vi "LEDS Controller.vi"(8 "error in":errorcluster) -> ()   [LabVIEW 2019]
doc: "This VI executes continuously carrying out the current operation and responding to updates or new operations. It will often contain the timing or control code that is difficult to place directly in TeleOp. This VI generally opens all sensors and motors and isolates the rest of the robot code from knowing how the operations are carried out."
uses:
  <vilib>/Rock Robotics/WPI/Framework/Completion Status.ctl
  LEDS Setpoints.ctl
  LEDS Operations.ctl
  <vilib>/Rock Robotics/SystemInterfaces/DIO/FPGA_DIOPWMChannel.ctl
  <vilib>/Rock Robotics/WPI/MotorControl/WPI_MotorControlOpen SPARK.vi
  <vilib>/Rock Robotics/Network Tables/NT Write Boolean.vi
panel:
  in  "Numeric":dbl=50.0
  in  "Interactive Values":T1={"Operation"=enum."Seizure-inducing", "Setpoint"=0.0, "Duration"=0.0, "seizure active"=FALSE, "pwmOutput"=0.0}
  out "Current\nCmd":string="Started at  17:26:23.947\n: Seizure-inducing,  S 0.0, D 0.000000"
  in  "Buttons":cluster{"Execute Cmd":bool, "Abort Cmd":bool}
  out "Command Timing":cluster{"Start Time (ms)":u32, "Iterations":i32}={"Start Time (ms)"=5015241, "Iterations"=0}
  out "Status":T3
  # "Tip: It may be helpful to observe inputs and sensor values.\nYou may also want to display tuning or debugging controls."
  # "Interactive Command: You may fill in the settings for a command\nand schedule it with the Execute button. You can observe and abort\nany command while fine tuning the code for the controller."
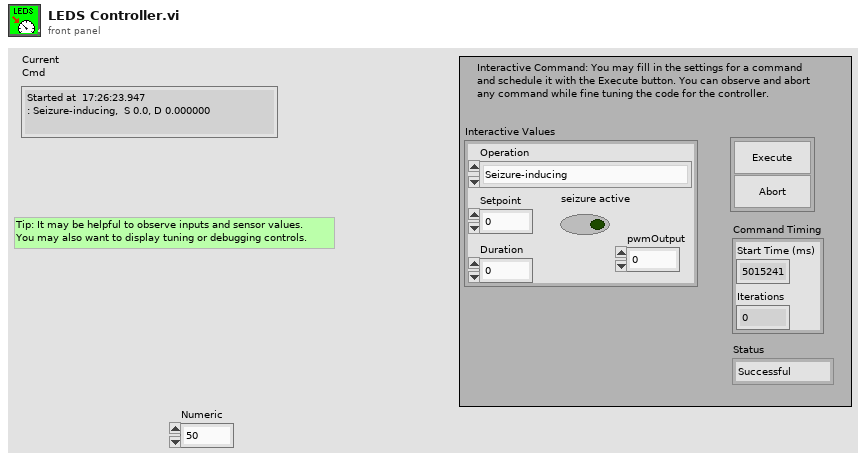
[diagram p1: front panel]
types:
  T1 = typedef "LEDS Setpoints.ctl" = cluster{"Operation":T2, "Setpoint":dbl, "Duration":dbl, "seizure active":bool, "pwmOutput":dbl}
  T2 = typedef "LEDS Operations.ctl" = enum16{"Reserve", "Read Current", "Immediate", "Seizure-inducing"}
  T3 = typedef "Completion Status.ctl" = enum16{"Successful", "Aborted", "Incomplete"}
  T4 = typedef "FPGA_DIOPWMChannel.ctl" = enum8{"PWM 0", "PWM 1", "PWM 2", "PWM 3", "PWM 4", "PWM 5", "PWM 6", "PWM 7", "PWM 8", "PWM 9", "PWM MXP 0", "PWM MXP 1", "PWM MXP 2", "PWM MXP 3", "PWM MXP 4", "PWM MXP 5", "PWM MXP 6", "PWM MXP 7", "PWM MXP 8", "PWM MXP 9", "Invalid"}
  T5 = typedef "WPI_MotorControlDeviceRef.ctl" = cluster{"DeviceStatus":errorcluster, "Type":T6, "PWM":cluster{"PWM Channel":T4, "DeadBand":T7}, "CAN":cluster{"Device Number":u8, "SetOutput VI Ref":variant, "GetOutput VI Ref":variant, "Enable VI Ref":variant, "Disable VI Ref":variant, "Data":variant}, "Invert":bool, "DIO PWM":cluster{"PWM \"Enable\" Channel":T4, "DIOChannel":T8, "PWM Rate":dbl}}
  T6 = typedef "WPI_MotorControlType.ctl" = enum16{"PWM", "CAN", "DIO PWM"}
  T7 = typedef "WPI_PWMDeadband.ctl" = cluster{"Name":string, "maxPositivePwm":i32, "minPositivePwm":i32, "centerPwm":i32, "maxNegativePwm":i32, "minNegativePwm":i32, "angularRange":u16}
  T8 = typedef "FPGA_DIOChannel.ctl" = enum8{"DIO 0", "DIO 1", "DIO 2", "DIO 3", "DIO 4", "DIO 5", "DIO 6", "DIO 7", "DIO 8", "DIO 9", "DIO MXP 0", "DIO MXP 1", "DIO MXP 2", "DIO MXP 3", "DIO MXP 4", "DIO MXP 5", "DIO MXP 6", "DIO MXP 7", "DIO MXP 8", "DIO MXP 9", "DIO MXP 10", "DIO MXP 11", "DIO MXP 12", "DIO MXP 13", "DIO MXP 14", "DIO MXP 15", "SPI Port CS1", "SPI Port CS2", "SPI Port CS3", "SPI Port MISO", "SPI Port MOSI", "Invalid"}
  T9 = typedef "Command Status Info.ctl" = cluster{"Name":string, "Status":T3, "notifier out":T10}
  T10 = typedef "Completion Notifier.ctl" = refnum<notifier>
  T11 = cluster{"Current Command":T1, "Command Timing":cluster{"Start Time (ms)":u32, "Iterations":i32}, "Command Arguments":cluster{"Command Info":T9, "Description":string, "Default Command":T1, "queue out":refnum<queue>, "Subsystem Name":string}}
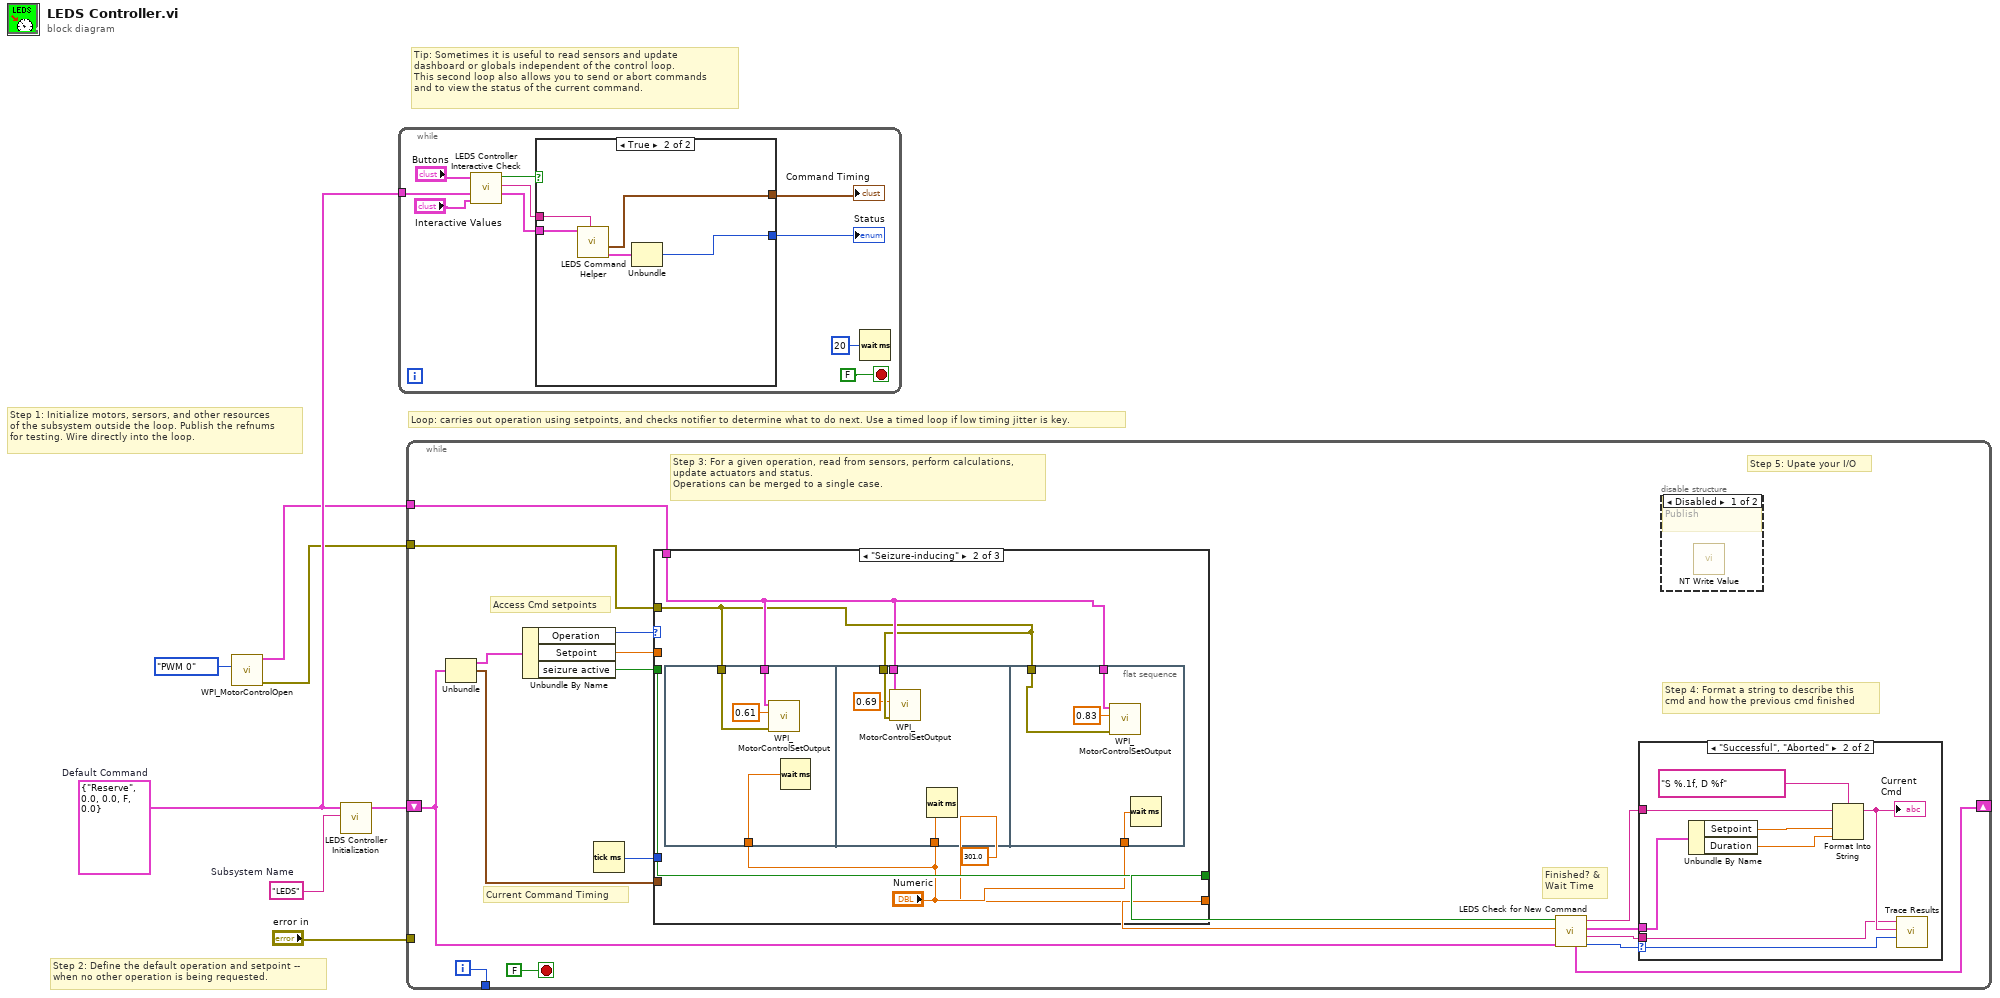
[diagram p0: block diagram]
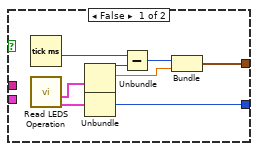
[diagram p2: hidden frame]
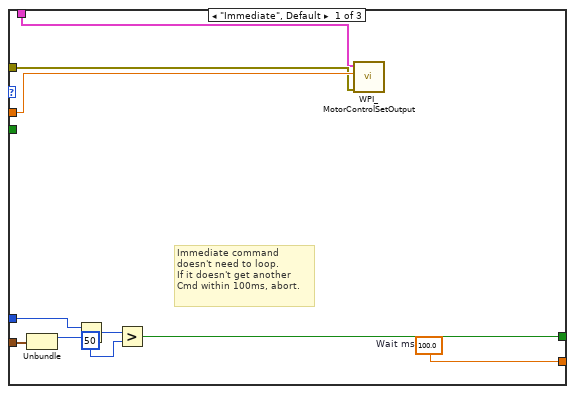
[diagram p5: hidden frame]
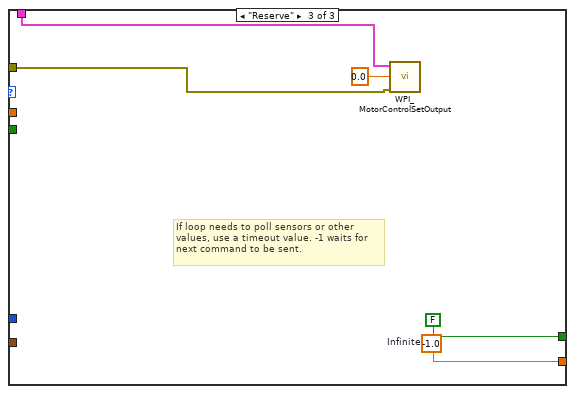
[diagram p6: hidden frame]
diagram:
  w4 = T1 {"Operation"=enum."Reserve", "Setpoint"=0.0, "Duration"=0.0, "seizure active"=FALSE, "pwmOutput"=0.0}  # Default Command
  w5 = "LEDS"  # Subsystem Name
  # "Tip: Sometimes it is useful to read sensors and update\ndashboard or globals independent of the control loop.\nThis second loop also allows you to send or abort commands\nand to view the status of the current command."
  # "Step 2: Define the default operation and setpoint --\nwhen no other operation is being requested."
  # "Step 1: Initialize motors, sersors, and other resources\nof the subsystem outside the loop. Publish the refnums\nfor testing. Wire directly into the loop."
  # "Loop: carries out operation using setpoints, and checks notifier to determine what to do next. Use a timed loop if low timing jitter is key."
  n1 = call-poly <vilib>:"WPI_MotorControlOpen.vi"("PWM Channel"=FPGA_DIOPWMChannel."PWM 0") -> ("error out"=w1:errorcluster, "MotorControlDeviceRef"=w2:T5)  [unwired: 9 in]
  n2 = call "LEDS Controller Initialization.vi"("Subsystem Name"=w5, "Default Command"=w4) -> ("Current Command"=w6:T11)  [unwired: 9 in]
  n3 = while {
    tunnel: w4 -> [w14]
    stop <- FALSE stop-if-true
    n4 = call "LEDS Controller Interactive Check.vi"("Interactive Command in"="Interactive Values", "Default Command"=w14, "Buttons"="Buttons") -> ("Interactive Command out"=w11:T1, "Trace String"=w12:string, "Schedule"=w13:bool)  [unwired: 6 in]
    n5 = case shown="True" w13 {
      tunnel: [w25 w30] -> w10
      tunnel: w11 -> [_ w28]
      tunnel: [w21 w26] -> w9
      tunnel: w12 -> [_ w29]
      frame False {
        n6 = Tick Count (ms)() -> (millisecond timer value=w20:u32)
        n7 = call "Read LEDS Operation.vi"() -> ("Command Info"=w18:T9, "SubSystem Data"=w19:T1)  [unwired: 9 in, 1 out]
        n8 = Unbundle(w19) -> ("Operation"=w24:T2, "Setpoint"=w22:dbl)  [unwired: 3 out]
        n9 = Unbundle(w18) -> ("Status"=w25:T3)  [unwired: 2 out]
        n10 = Subtract(x=w20, y=w24) -> (x-y=w23:u32)
        n11 = Bundle(w23, "Setpoint"=w22) -> (w21:cluster{u32, "Setpoint":dbl})  [unwired: 1 in]
      }
      frame True {
        n12 = call "LEDS Command Helper.vi"("Description"=w29, "SubSystem Data"=w28) -> ("Command Info Out"=w27:T9, "Command Timing"=w26:cluster{"Start Time (ms)":u32, "Iterations":i32})  [unwired: 7 in, 1 out]
        n13 = Unbundle(w27) -> ("Status"=w30:T3)  [unwired: 2 out]
      }
    }
    "Status" <- w10
    "Command Timing" <- w9
    n14 = Wait (ms)(milliseconds to wait=u32 20) -> ()  [unwired: 1 out]
  }
  n15 = while {
    shift-right: [w41] -> _
    shift-left: w6 -> [w34]
    tunnel: [w47] -> _
    tunnel: "error in" -> [_]
    tunnel: w2 -> [w31]
    tunnel: w1 -> [w32]
    i -> [w47]
    stop <- FALSE stop-if-true
    # "Step 5: Upate your I/O"
    # "Step 4: Format a string to describe this\ncmd and how the previous cmd finished"
    # "Current Command Timing"
    # "Access Cmd setpoints"
    # "Finished? &\nWait Time"
    # "Step 3: For a given operation, read from sensors, perform calculations,\nupdate actuators and status.\nOperations can be merged to a single case."
    n16 = Unbundle(w34) -> ("Current Command"=w46:T1, "Command Timing"=w42:cluster{"Start Time (ms)":u32, "Iterations":i32})  [unwired: 1 out]
    n17 = Unbundle By Name(w46) -> ("Operation"=w45:T2, "Setpoint"=w44:dbl, "seizure active"=w33:bool)
    n18 = Tick Count (ms)() -> (millisecond timer value=w43:u32)
    n19 = case shown="\"Seizure-inducing\"" w45 {
      tunnel: [w66 301.0 ("Infinite") w88] -> w39
      tunnel: [w60 w71 FALSE ("ignore previous (F)")] -> w40
      tunnel: w42 -> [w62 _ _]
      tunnel: w44 -> [w59 _ _]
      tunnel: w43 -> [w61 _ _]
      tunnel: w33 -> [_ w71 _]
      tunnel: w32 -> [w58 w67 w84]
      tunnel: w31 -> [w57 w68 w85]
      frame "Immediate", Default {
        w66 = 100.0  # Wait ms
        # "Immediate command\ndoesn't need to loop.\nIf it doesn't get another\nCmd within 100ms, abort."
        n20 = Unbundle(w62) -> ("Start Time (ms)"=w65:u32)  [unwired: 1 out]
        n21 = Subtract(x=w61, y=w65) -> (x-y=w64:u32)
        n22 = Greater?(x=w64, y=u8 50 ("Left Motor")) -> (0:w60:bool)
        n23 = call <vilib>:"WPI_MotorControlSetOutput.vi"("error in (no error)"=w58, "Output"=w59, "MotorControlDevRef"=w57) -> ()  [unwired: 6 in, 3 out]
      }
      frame "Seizure-inducing" {
        n24 = flat-sequence {
          tunnel: w68 -> [w75]
          tunnel: w67 -> [w74]
          tunnel: "Numeric" -> [w72]
          tunnel: w67 -> [w79]
          tunnel: w68 -> [w77]
          tunnel: "Numeric" -> [w76]
          tunnel: w67 -> [w82]
          tunnel: w68 -> [w81]
          tunnel: "Numeric" -> [w80]
          frame #0 {
            n25 = call <vilib>:"WPI_MotorControlSetOutput.vi"("error in (no error)"=w74, "Output"=0.61, "MotorControlDevRef"=w75) -> ()  [unwired: 6 in, 3 out]
            n26 = Wait (ms)(milliseconds to wait=w72) -> ()  [unwired: 1 out]
          }
          frame #1 {
            n27 = call <vilib>:"WPI_MotorControlSetOutput.vi"("error in (no error)"=w79, "Output"=0.69, "MotorControlDevRef"=w77) -> ()  [unwired: 6 in, 3 out]
            n28 = Wait (ms)(milliseconds to wait=w76) -> ()  [unwired: 1 out]
          }
          frame #2 {
            n29 = call <vilib>:"WPI_MotorControlSetOutput.vi"("error in (no error)"=w82, "Output"=0.83, "MotorControlDevRef"=w81) -> ()  [unwired: 6 in, 3 out]
            n30 = Wait (ms)(milliseconds to wait=w80) -> ()  [unwired: 1 out]
          }
        }
      }
      frame "Reserve" {
        w88 = -1.0  # Infinite
        # "If loop needs to poll sensors or other\nvalues, use a timeout value. -1 waits for\nnext command to be sent."
        n31 = call <vilib>:"WPI_MotorControlSetOutput.vi"("error in (no error)"=w84, "Output"=0.0, "MotorControlDevRef"=w85) -> ()  [unwired: 6 in, 3 out]
      }
    }
    n32 = call "LEDS Check for New Command.vi"("Current Command"=w34, "Wait time (ms)"=w39, "Finished?"=w40) -> ("Completion"=w35:T3, "Subsystem Name"=w36:string, "Current Command"=w37:T1, "Initial Trace String"=w38:string, "NextCommand"=w41:T11)  [unwired: 4 in]
    n33 = case shown="\"Successful\", \"Aborted\"" w35 {
      selector: w35 -> [_ w56]
      tunnel: w38 -> [_ w52]
      tunnel: w37 -> [_ w53]
      tunnel: w36 -> [_ w49]
      frame "Incomplete", Default {
        # "Continuing current command"
      }
      frame "Successful", "Aborted" {
        # "Report and setup for next command"
        n34 = Unbundle By Name(w53) -> ("Setpoint"=w55:dbl, "Duration"=w50:dbl)
        n35 = Format Into String(format string="S %.1f, D %f", initial string=w52, w55, w50) -> (resulting string=w51:string)  [unwired: 1 in, 1 out]
        "Current\nCmd" <- w51
        n36 = call <vilib>:"Trace Results.vi"("Status of previous command"=w56, "Description"=w51, "Subsystem"=w49) -> ()  [unwired: 9 in]
      }
    }
    n37 = disable-structure shown="Disabled" {
      frame Disabled {
        # "Publish"
        n38 = call-poly <vilib>:"NT Write Value.vi"() -> ()  [unwired: 11 in, 1 out]
      }
      frame Enabled {
      }
    }
  }
